vi "Read View.vi"(8 "error in (no error)":errorcluster, 11 "View Test In":refnum<class "View Dev Test.lvclass">) -> (0 "error out":errorcluster, 2 "View":refnum<class "View.lvclass">, 3 "View Test Out":refnum<class "View Dev Test.lvclass">)   [LabVIEW 2020, in "View Dev Test.lvclass"]
uses:
  View Dev Test.lvclass
  source/Framework/View/View.lvclass
  C:/Git/astemes-triarc-framework/source/Framework Test/Base Class Test/Base Test.lvclass
  source/Framework Test Suite/Base Class Test/Base Test.lvclass/Base Test.ctl
  source/Framework/Base/Base.lvclass
  View Dev Test.lvclass/View Dev Test.ctl
  source/Framework Test Suite/Base Class Test/Base Test.lvclass
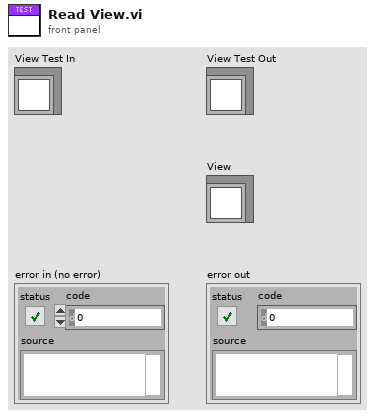
[diagram p1: front panel]
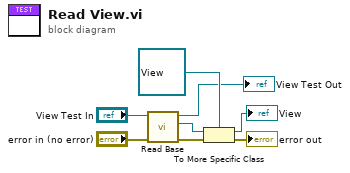
[diagram p0: block diagram]
diagram:
  n1 = call "Read Base.vi"("error in (no error)"="error in (no error)", "Base Class Test In"="View Test In") -> ("error out"=w5:errorcluster, "Base.lvclass"=w4:refnum<class "Base.lvclass">, "Base Class Test Out"=→"View Test Out":refnum<class "View Dev Test.lvclass">)  [unwired: 7 in]
  n2 = To More Specific Class(target class=refnum<class "View.lvclass"> refnum ("UI View.lvclass"), reference=w4, error in=w5) -> (specific class reference=→"View":refnum<class "View.lvclass">, error out=→"error out":errorcluster)
